vi "practica11RNA.vi"(6 "b":dbl, 10 "w":dbl[](array[numeric]), 11 "x":dbl[](array[numeric])) -> (3 "a":dbl)   [LabVIEW 2017]
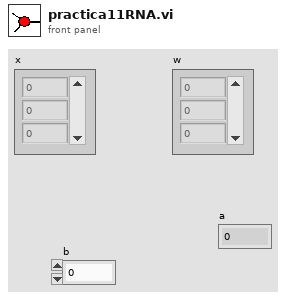
[diagram p1: front panel]
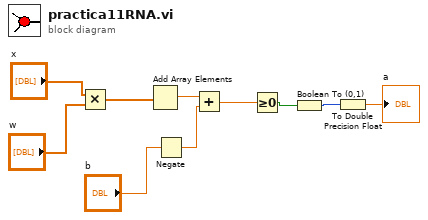
[diagram p0: block diagram]
diagram:
  n1 = Multiply(x="x", y="w") -> (x*y=w8:dbl[])
  n2 = Add Array Elements(numeric array=w8) -> (sum=w7:dbl)
  n3 = Negate(x="b") -> (-x=w6:dbl)
  n4 = Add(x=w7, y=w6) -> (x+y=w4:dbl)
  n5 = Greater Or Equal To 0?(x=w4) -> (x >= 0?=w3:bool)
  n6 = Boolean To (0,1)(Boolean=w3) -> (0, 1=w2:i16)
  n7 = To Double Precision Float(number=w2) -> (double precision float=→"a":dbl)
